vi "FPGA Measurement for Protection.vi"(0 "resampled data":T5, 1 "number of channels":T4=1 items=["1"=1, "2"=2, "3"=3, "4"=4, "5"=5, "6"=6, "7"=7, "8"=8, "9"=9, "10"=10, "11"=11, "12"=12, "13"=13, "14"=14, "15"=15, "16"=16], 5 "resampling info":T3={"nominal frequency"=enum."50 Hz", "resampling valid?"=FALSE, "samples per cycle"=192}, 9 "input valid? (T)":bool=TRUE, 12 "ready for output? (T)":bool=TRUE) -> (4 "output phasor":T1 {"phasor timestamp [s]" format="%#.6g"; "phase [pi]" format="%#.6g"}, 6 "output frequency":T2 {"frequency timestamp [s]" format="%#.6g"}, 10 "output valid?":bool, 14 "ready for input?":bool, 15 "error":i32)   [LabVIEW 2013, in "NI_EP_Protection_FPGA.lvlib"]
doc: "Computes the instantaneous magnitude, phase, and frequency values of the fundamental frequency component for protection applications. The output rate is 24 samples per cycle. You must use the FPGA Resampling VI to resample even-time-spaced voltage and current signals into even-angle-spaced signals before running this VI."
uses:
  <vilib>/addons/Electrical Power/Protection/NI_EP_Protection_FPGA.lvlib
  <vilib>/addons/Electrical Power/PQ/Resampling/FPGA/subVIs/fpga_Resampled.ctl
  <vilib>/addons/Electrical Power/PQ/Resampling/FPGA/subVIs/fpga_NofCH.ctl
  <vilib>/addons/Electrical Power/PQ/Resampling/FPGA/subVIs/fpga_Resampling Info.ctl
  <vilib>/addons/Electrical Power/Protection/Protection Measurement/subVIs/fpga_OutputFrequency.ctl
  <vilib>/addons/Electrical Power/Protection/Protection Measurement/subVIs/fpga_OutputMagPhase.ctl
  <vilib>/addons/Electrical Power/PQ/Resampling/NI_EP_Resample_FPGA.lvlib
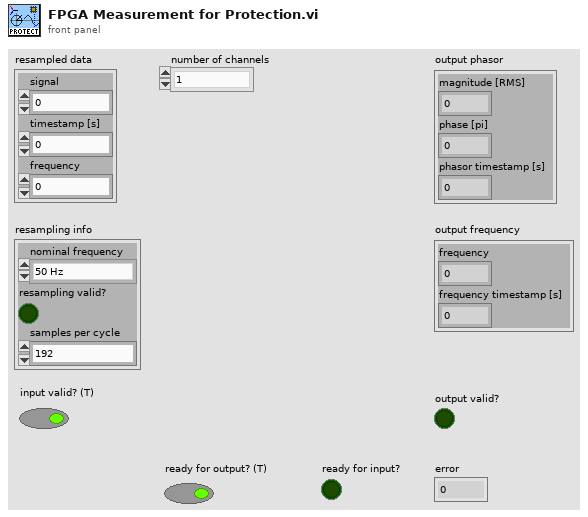
[diagram p1: front panel]
types:
  T1 = typedef "NI_EP_Protection_FPGA.lvlib/fpga_OutputMagPhase.ctl" = cluster{"magnitude [RMS]":fxp<+,32,6>, "phase [pi]":fxp<+/-,32,2>, "phasor timestamp [s]":fxp<+,64,32>}
  T2 = typedef "NI_EP_Protection_FPGA.lvlib/fpga_OutputFrequency.ctl" = cluster{"frequency":fxp<+,32,8>, "frequency timestamp [s]":fxp<+,64,32>}
  T3 = typedef "NI_EP_Resample_FPGA.lvlib/fpga_Resampling Info.ctl" = cluster{"nominal frequency":enum16{"50 Hz", "60 Hz"}, "resampling valid?":bool, "samples per cycle":u16}
  T4 = typedef "NI_EP_Resample_FPGA.lvlib/fpga_NofCH.ctl" = u8
  T5 = typedef "NI_EP_Resample_FPGA.lvlib/fpga_Resampled.ctl" = cluster{"signal":fxp<+/-,32,3>, "timestamp [s]":fxp<+,64,32>, "frequency":fxp<+,32,8>}
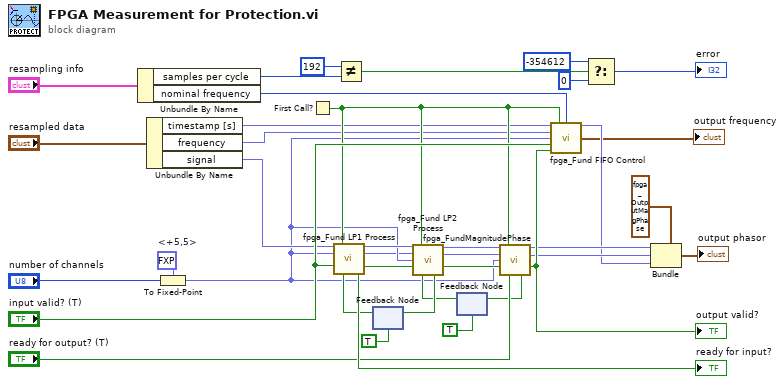
[diagram p0: block diagram]
diagram:
  w16 = fxp<+,5,5> 0.0  # <+5,5>
  n1 = Unbundle By Name("resampling info") -> ("samples per cycle"=w10:u16, "nominal frequency"=w11:enum16{"50 Hz", "60 Hz"})
  n2 = Unbundle By Name("resampled data") -> ("timestamp [s]"=w19:fxp<+,64,32>, "frequency"=w17:fxp<+,32,8>, "signal"=w18:fxp<+/-,32,3>)
  n3 = To Fixed-Point(fixed-point type=w16, number="number of channels") -> (fixed-point=w15:fxp<+,5,5>)
  n4 = First Call?() -> (First Call?: T/F=w20:bool)
  n5 = Not Equal?(x=u16 192, y=w10) -> (x != y?=w8:bool)
  n6 = feedback #1(TRUE ("ready for input")) -> (w29:bool)
  n7 = call <vilib>:"fpga_Fund LP1 Process.vi"("input data"=w18, "reset"=w20, "Ch"=w15, "input valid"="input valid? (T)", "ready for output"=w29) -> ("re"=w31:fxp<+/-,32,5>, "im"=w1:fxp<+/-,32,5>, "output valid"=w28:bool, "ready for input"=→"ready for input?":bool)  [unwired: 7 in]
  n8 = feedback #2(TRUE ("ready for input")) -> (w22:bool)
  n9 = call <vilib>:"fpga_Fund LP2 Process.vi"("re"=w31, "reset"=w20, "im"=w1, "#Ch"=w15, "input valid"=w28, "ready for output"=w22) -> ("re filtered"=w26:fxp<+/-,32,6>, "im filtered"=w25:fxp<+/-,32,6>, "output valid"=w24:bool, "ready for input"=w30:bool)  [unwired: 6 in]
  n10 = feedback-in #1(w30) -> ()
  n11 = call <vilib>:"fpga_FundMagnitudePhase.vi"("re"=w26, "reset"=w20, "im"=w25, "Ch"=w15, "input valid"=w24, "ready for output"="ready for output? (T)") -> ("rms magnitude"=w14:fxp<+,32,6>, "phase"=w13:fxp<+/-,32,2>, "output valid"=w35:bool, "ready for input"=w23:bool)  [unwired: 6 in]
  "output valid?" <- w35
  n12 = feedback-in #2(w23) -> ()
  n13 = call <vilib>:"fpga_Fund FIFO Control.vi"("Time stamp"=w19, "reset"=w20, "nominal frequency"=w11, "Frequency"=w17, "#ch"=w15, "PMU VI input valid"="input valid? (T)", "PMU VI output valid"=w35) -> ("Time Stamp out"=w12:fxp<+,64,32>, "output frequency"=→"output frequency":T2)  [unwired: 7 in]
  n14 = Select(t=-354612 ("error"), s=w8, f=0) -> (s? t:f=→"error":i32)
  n15 = Bundle(cluster=T1 {"magnitude [RMS]"=0.0, "phase [pi]"=0.0, "phasor timestamp [s]"=0.0} ("output data"), "magnitude [RMS]"=w14, "phase [pi]"=w13, "phasor timestamp [s]"=w12) -> (→"output phasor":T1)
